vi "Write cluster.vi"(10 "cluster":T1, 11 "ValveModbus in":refnum<class "NeedleValve.lvclass">) -> (3 "ValveModbus out":refnum<class "NeedleValve.lvclass">)   [LabVIEW 2019, in "NeedleValve.lvclass"]
uses:
  NeedleValve.lvclass
  modbus engine custom/MB_ENGINE_class/Settings.ctl
  modbus engine custom/MB_ENGINE_class/MB_ENGINE.lvclass
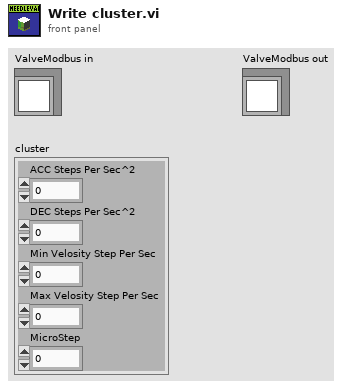
[diagram p1: front panel]
types:
  T1 = typedef "MB_ENGINE.lvclass/Settings.ctl" = cluster{"ACC Steps Per Sec^2":u16, "DEC Steps Per Sec^2":u16, "Min Velosity Step Per Sec":u16, "Max Velosity Step Per Sec":u16, "MicroStep":u16}
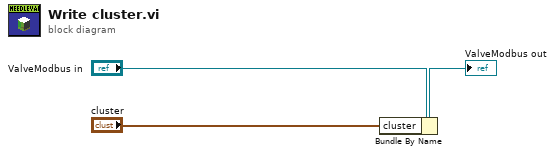
[diagram p0: block diagram]
diagram:
  n1 = Bundle By Name(cluster="ValveModbus in", "cluster"="cluster") -> (→"ValveModbus out":refnum<class "NeedleValve.lvclass">)
